vi "Read Spectrum Reader.vi"(8 "error in (no error)":errorcluster, 11 "Refnum in":refnum<k21>) -> (0 "error out":errorcluster, 2 "Boolean":bool, 3 "output waveform":waveform(dbl))   [LabVIEW 2017]
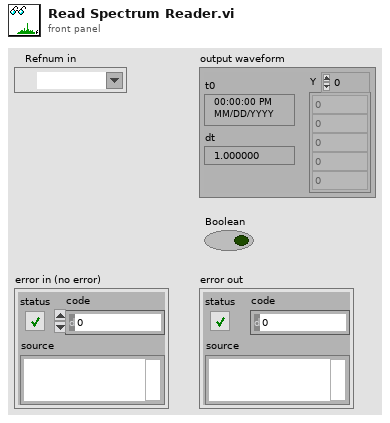
[diagram p1: front panel]
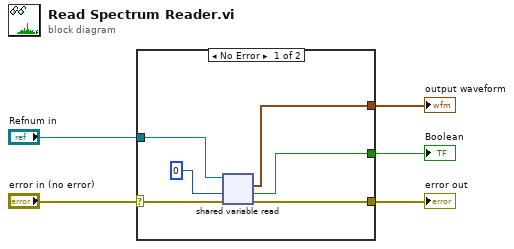
[diagram p0: block diagram]
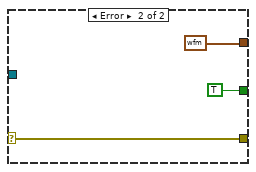
[diagram p2: hidden frame]
diagram:
  n1 = case shown="No Error" "error in (no error)" {
    selector: "error in (no error)" -> [w6 w14]
    tunnel: [w11 waveform(dbl) {"t0"=timestamp(0 s since 1904-01-01), "dt"=1.0, "Y"=[]} ("output waveform")] -> w5
    tunnel: [w10 w14] -> w4
    tunnel: [w9 TRUE] -> w3
    tunnel: "Refnum in" -> [w7 _]
    frame No Error {
      n2 = shared-variable-read(w7, w6, 0 ("timeout ms (-1)")) -> (w10:errorcluster, w9:bool, w11:waveform(dbl))  [unwired: 1 out]
    }
    frame Error {
    }
  }
  "output waveform" <- w5
  "error out" <- w4
  "Boolean" <- w3
